vi "svx_Polar_Cal_ScaleMaximum.vi"(10 "scale width":dbl, 11 "original maximum":dbl) -> (3 "best maximum":dbl)   [LabVIEW 2017, in "SVX Polar Plot.xctl"]
uses:
  <vilib>/addons/_XControls/Polar Plot/SVX Polar Plot.xctl
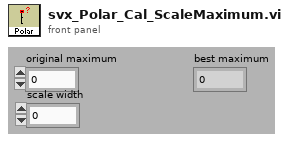
[diagram p1: front panel]
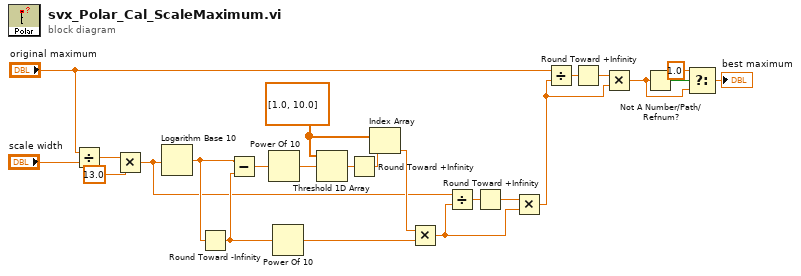
[diagram p0: block diagram]
diagram:
  w16 = dbl[] [1.0, 10.0] ("array")
  n1 = Divide(x="original maximum", y="scale width") -> (x/y=w12:dbl)
  n2 = Multiply(x=w12, y=13.0) -> (x*y=w10:dbl)
  n3 = Logarithm Base 10(1:w10) -> (0:w18:dbl)
  n4 = Round Toward -Infinity(1:w18) -> (0:w17:dbl)
  n5 = Subtract(x=w18, y=w17) -> (x-y=w19:dbl)
  n6 = Power Of 10(x=w19) -> (10^x=w20:dbl)
  n7 = Power Of 10(x=w17) -> (10^x=w15:dbl)
  n8 = Threshold 1D Array(2:w20, 3:w16) -> (0:w21:dbl)  [unwired: 1 in]
  n9 = Round Toward +Infinity(x=w21) -> (ceil(x): smallest int >= x=w22:dbl)
  n10 = Index Array(array=w16, index=w22) -> (element=w14:dbl)
  n11 = Multiply(x=w14, y=w15) -> (x*y=w13:dbl)
  n12 = Divide(x=w10, y=w13) -> (x/y=w24:dbl)
  n13 = Round Toward +Infinity(x=w24) -> (ceil(x): smallest int >= x=w23:dbl)
  n14 = Multiply(x=w23, y=w13) -> (x*y=w7:dbl)
  n15 = Divide(x="original maximum", y=w7) -> (x/y=w9:dbl)
  n16 = Round Toward +Infinity(x=w9) -> (ceil(x): smallest int >= x=w8:dbl)
  n17 = Multiply(x=w8, y=w7) -> (x*y=w2:dbl)
  n18 = Not A Number/Path/Refnum?(number/path/refnum=w2) -> (NaN/Path/Refnum?=w4:bool)
  n19 = Select(t=1.0, s=w4, f=w2) -> (s? t:f=→"best maximum":dbl)
